vi "6D_Global.vi"() -> ()   [LabVIEW 2022 SP3]
panel:
  in  "Start Log":bool
  in  "Stop Log":bool
  in  "Trigger":timestamp
  out "RUN ACK 2":bool
  out "RUN ACK":bool
  out "Device information 2":string[](array[string])
  out "Device information":string[](array[string])
  in  "PPSU IP 2":u8[](array[numeric])=[169, 254, 146, 100]
  out "No.of slaves 2":u8
  in  "T-Power 2":string
  in  "T-Current 2":string
  in  "T-Voltage 2":string
  in  "Drive Config":path
  out "No.of slaves":u8
  in  "T-Power":string
  in  "T-Current":string
  in  "T-Voltage":string
  in  "PPSU IP":u8[](array[numeric])=[0, 0, 0, 0]
  in  "DO  Configuration":cluster{"NAME":string, "lines":tag}[](array[cluster])=[{"NAME"="LOX GD COM", "lines"="cDAQ9185-1E540F5Mod1/port0/line0"}, {"NAME"="ATF GD COM", "lines"="cDAQ9185-1E540F5Mod1/port0/line1"}]
  out "DO Com":bool[](array[boolean])
  out "Stop DAQ":bool
  out "Start DAQ":bool
  out "Datalog Prefix":string
  out "Contineous":bool
  in  "Log Period":dbl=900.0
  out "Exit":bool
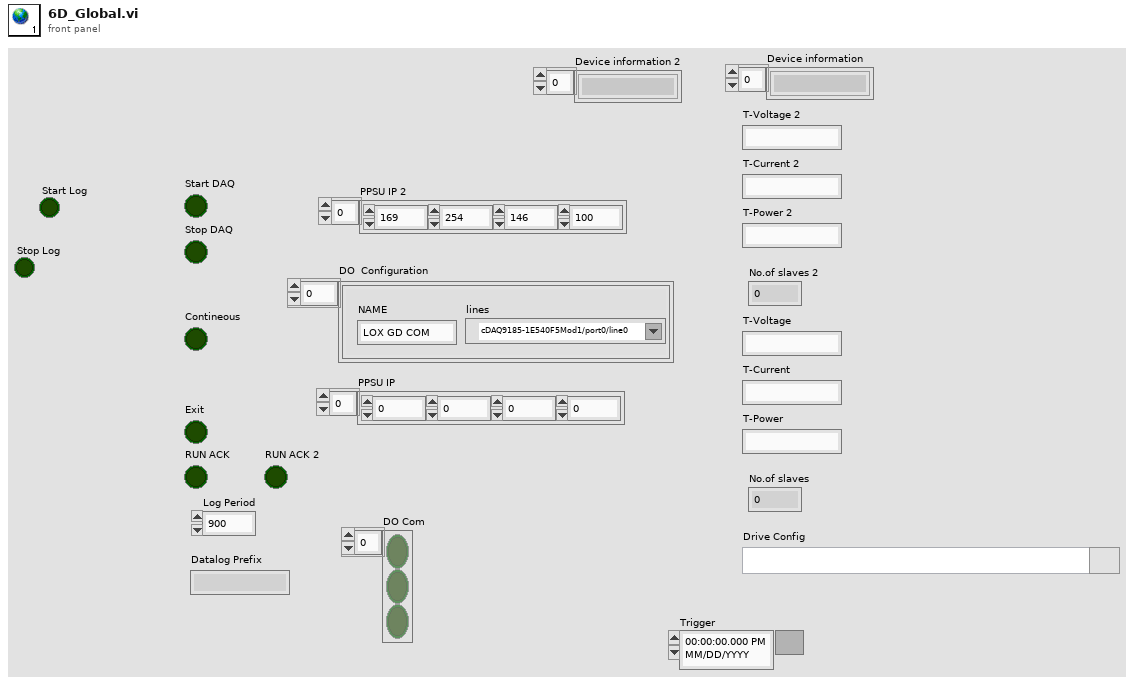
[diagram p1: front panel]
diagram:
